vi "Write Setup File.lvclass.vi"(8 "error in (no error)":errorcluster, 10 "Setup File.lvclass":refnum<class "Setup File.lvclass">, 11 "SPARC4_AC in":refnum<class "S4GUI.lvclass">) -> (0 "error out":errorcluster, 3 "SPARC4_AC out":refnum<class "S4GUI.lvclass">)   [LabVIEW 2018, in "S4GUI.lvclass"]
uses:
  S4GUI.lvclass
  SetupFile/Setup File.lvclass
  S4GUI.lvclass/S4GUI.ctl
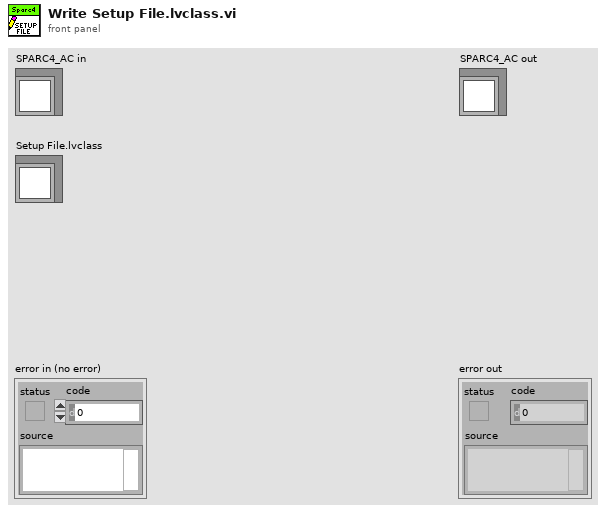
[diagram p1: front panel]
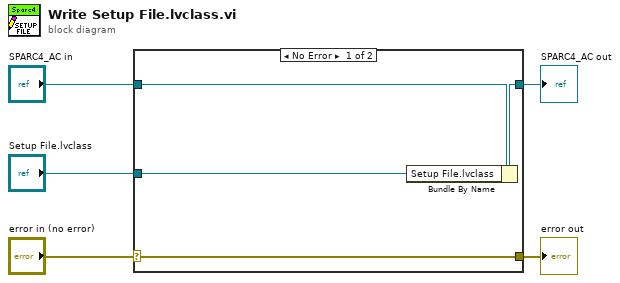
[diagram p0: block diagram]
diagram:
  n1 = case shown="No Error" "error in (no error)" {
    selector: "error in (no error)" -> [w9 w10]
    tunnel: [w9 w10] -> w4
    tunnel: [w7 w11] -> w2
    tunnel: "SPARC4_AC in" -> [w8 w11]
    tunnel: "Setup File.lvclass" -> [w6 _]
    frame No Error {
      n2 = Bundle By Name(cluster=w8, "Setup File.lvclass"=w6) -> (w7:refnum<class "S4GUI.lvclass">)
    }
    frame Error {
    }
  }
  "error out" <- w4
  "SPARC4_AC out" <- w2
